vi "Append Table to Document.vi"(0 "PDF Report IN":refnum<class "PDF Report Class.lvclass">, 1 "Table properties":T18={"Table position"=1, "SpacingBefore (points)"=12.0, "SpacingAfter (points)"=12.0} {"Table position" items=["LEFT", "CENTER", "RIGHT"]}, 3 "Row background color":T20={"color"=16777225, "at each"=0}, 7 "PDF Table":refnum<class "Pdfp Table Class.lvclass">, 9 "Caption":string, 11 "error in (no error)":errorcluster, 12 "Row  [ ]":T1) -> (4 "PDF Report OUT":refnum<class "PDF Report Class.lvclass">, 15 "error out":errorcluster)   [LabVIEW 2019]
doc: "<B>ENGLISH</B>\nAppends a table to the PDF document.\n\n<B>FRANÇAIS</B>\nAjoute un tableau au document PDF.\n\nVersion 2.0\nDeveloped by Jean-Marc Simard\nCopyright © 2012, Exaprom Inc.\nAll rights reserved.\nLicense: BSD\n\nWith iTextSharp 4.1.6 (http://itextsharp.sourceforge.net)\nunder Mozilla Public License Version 1.1\n(http://www.mozilla.org/MPL/MPL-1.1.html)"
uses:
  <userlib>/Exaprom PDF/LV Class/PDF Report Class/PDF Report Class.lvclass
  <userlib>/Exaprom PDF/Controls/Table Controls/Row Back Ground color Datas.ctl
  <userlib>/Exaprom PDF/Controls/Table Controls/Table properties.ctl
  <userlib>/Exaprom PDF/Controls/Table Controls/Table position.ctl
  <userlib>/Exaprom PDF/LV Class/Pdfp Table Class/Pdfp Table Class.lvclass
  <userlib>/Exaprom PDF/Controls/Table Controls/Table Appearance and Font Row [ ].ctl
  <userlib>/Exaprom PDF/Controls/Table Controls/One Row Appearance.ctl
  <userlib>/Exaprom PDF/Controls/Table Controls/Row from to.ctl
  <userlib>/Exaprom PDF/Controls/Table Controls/Cell, Alignment, LS and Font - hide Vmerge.ctl
  <userlib>/Exaprom PDF/Controls/Table Controls/Cell Type, Alignment and LS.ctl
  <userlib>/Exaprom PDF/Controls/Table Controls/Cell Alignment 20px.ctl
  <userlib>/Exaprom PDF/Controls/Table Controls/Text vertical arrangement.ctl
  <userlib>/Exaprom PDF/Controls/Text Controls/Line spacing.ctl
  <userlib>/Exaprom PDF/Controls/Table Controls/Cell Appearance.ctl
  <userlib>/Exaprom PDF/Controls/Table Controls/Cell Border 20 px.ctl
  <userlib>/Exaprom PDF/Controls/Table Controls/Merge Horizontal.ctl
  <userlib>/Exaprom PDF/Controls/Table Controls/Merge Vertical.ctl
  <userlib>/Exaprom PDF/Controls/Font Controls/Font complete cluster.ctl
  <userlib>/Exaprom PDF/Controls/Font Controls/Font size.ctl
  <userlib>/Exaprom PDF/Controls/Font Controls/Font color.ctl
  <userlib>/Exaprom PDF/Controls/Font Controls/Type and encoding.ctl
  <userlib>/Exaprom PDF/Controls/Text Controls/Unicode/Type and run direction.ctl
  <userlib>/Exaprom PDF/Not  in the library/Images for controls/Image or Table.ctl
  C:/Program Files/National Instruments/LabVIEW 2019/user.lib/Exaprom PDF/DLL/itextsharp.dll
  DLL/itextsharp.dll
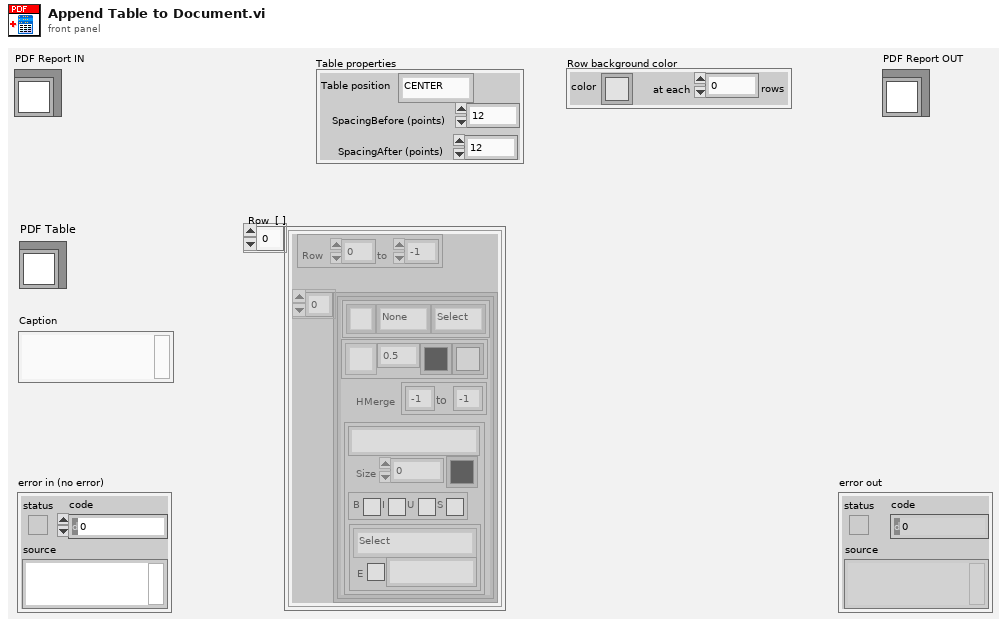
[diagram p1: front panel]
types:
  T1 = typedef "Table Appearance and Font Row [ ].ctl" = T2[]
  T2 = typedef "One Row Appearance.ctl" = cluster{"Row":T3, "Cell [ ]":T4[]}
  T3 = typedef "Row from to.ctl" = cluster{"From #":i16, "to #":i16}
  T4 = typedef "Cell, Alignment, LS and Font - hide Vmerge.ctl" = cluster{"Text":T5, "Cell Appearance":T9, "HMerge":T11, "VMerge":T12, "Font":T13}
  T5 = typedef "Cell Type, Alignment and LS.ctl" = cluster{"Cell Alignment":T6, "Text rotation":T7, "Line spacing":T8}
  T6 = typedef "Cell Alignment 20px.ctl" = u16
  T7 = typedef "Text vertical arrangement.ctl" = enum16{"None", "Clockwise", "Counterclockwise"}
  T8 = typedef "Line spacing.ctl" = enum16{"Select", "1.0", "1.5", "2.0"}
  T9 = typedef "Cell Appearance.ctl" = cluster{"Border":T10, "Thickness":sgl, "Color":u32, "BG":u32}
  T10 = typedef "Cell Border 20 px.ctl" = u16
  T11 = typedef "Merge Horizontal.ctl" = cluster{"From":i8, "to":i8}
  T12 = typedef "Merge Vertical.ctl" = cluster{"From":i8, "to":i8}
  T13 = typedef "Font complete cluster.ctl" = cluster{"Name":string, "Size":T14, "Color":T15, "Style":cluster{"Bold":bool, "Italic":bool, "Underline":bool, "Strikeout":bool}, "Type":T16}
  T14 = typedef "Font size.ctl" = sgl
  T15 = typedef "Font color.ctl" = u32
  T16 = typedef "Type and encoding.ctl" = cluster{"Type&direction":T17, "Embedded":bool, "Encoding":string}
  T17 = typedef "Type and run direction.ctl" = enum16{"Select", "ASCII", "UTF-16", "UTF-16 (default)", "UTF-16 (LTR)", "UTF-16 (RTL)"}
  T18 = typedef "Table properties.ctl" = cluster{"Table position":T19, "SpacingBefore (points)":sgl, "SpacingAfter (points)":sgl}
  T19 = typedef "Table position.ctl" = i32
  T20 = typedef "Row Back Ground color Datas.ctl" = cluster{"color":u32, "at each":i16}
  T21 = typedef "Image or Table.ctl" = enum16{"Image", "Table"}
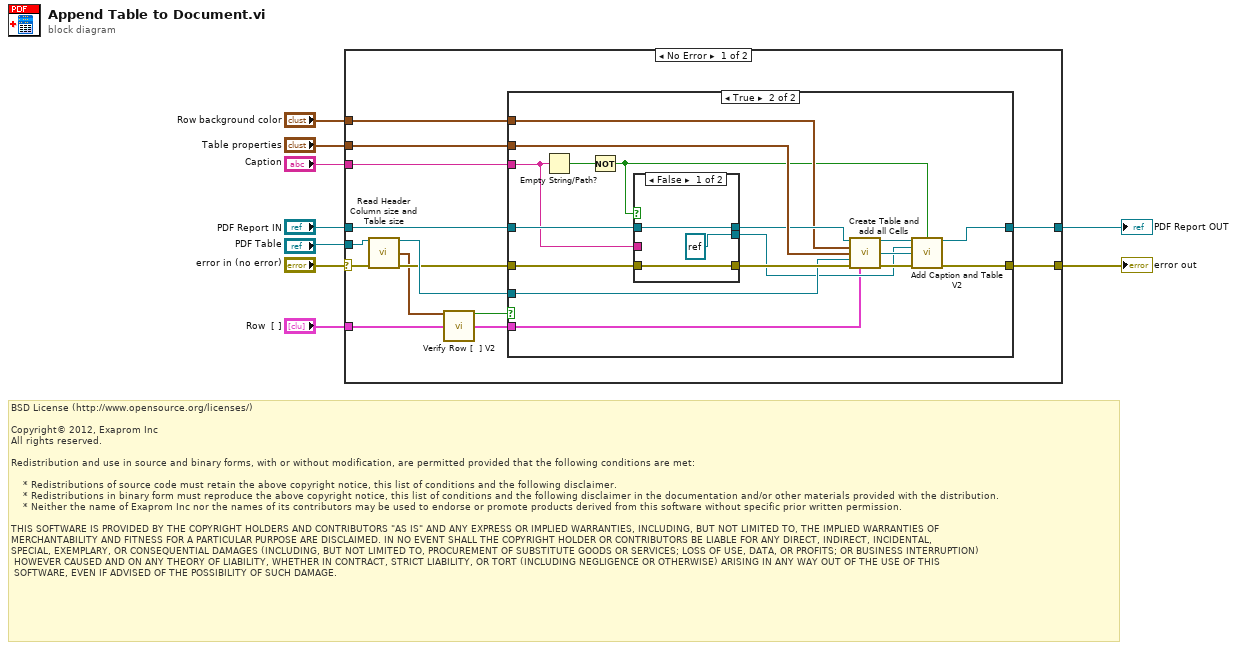
[diagram p0: block diagram]
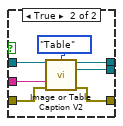
[diagram p3: hidden frame]
diagram:
  # "BSD License (http://www.opensource.org/licenses/)\n\nCopyright© 2012, Exaprom Inc\nAll rights reserved.\n\nRedistribution and use in source and binary forms, with or without modification, are permitted provided that the following conditions are met:\n\n    * Redistributions of source code must retain the above copyright notice, this list of conditions and the following disclaimer.\n    * Redistributions in binary form must reproduce the above copyright notice, this list of conditions and the following disclaimer in the documentation and/or other materials provided with the distribution.\n    * Neither the name of Exaprom Inc nor the names of its contributors may be used to endorse or promote products derived from this software without specific prior written permission.\n\nTHIS SOFTWARE IS PROVIDED BY THE COPYRIGHT HOLDERS AND CONTRIBUTORS \"AS IS\" AND ANY EXPRESS OR IMPLIED WARRANTIES, INCLUDING, BUT NOT LIMITED TO, THE IMPLIED WARRANTIES OF \nMERCHANTABILITY AND FITNESS FOR A PARTICULAR PURPOSE ARE DISCLAIMED. IN NO EVENT SHALL THE COPYRIGHT HOLDER OR CONTRIBUTORS BE LIABLE FOR ANY DIRECT, INDIRECT, INCIDENTAL,\nSPECIAL, EXEMPLARY, OR CONSEQUENTIAL DAMAGES (INCLUDING, BUT NOT LIMITED TO, PROCUREMENT OF SUBSTITUTE GOODS OR SERVICES; LOSS OF USE, DATA, OR PROFITS; OR BUSINESS INTERRUPTION)\n HOWEVER CAUSED AND ON ANY THEORY OF LIABILITY, WHETHER IN CONTRACT, STRICT LIABILITY, OR TORT (INCLUDING NEGLIGENCE OR OTHERWISE) ARISING IN ANY WAY OUT OF THE USE OF THIS\n SOFTWARE, EVEN IF ADVISED OF THE POSSIBILITY OF SUCH DAMAGE."
  n1 = case shown="No Error" "error in (no error)" {
    selector: "error in (no error)" -> [w17 w53]
    tunnel: "Table properties" -> [w22 _]
    tunnel: "PDF Report IN" -> [w23 w54]
    tunnel: "Caption" -> [w18 _]
    tunnel: "Row background color" -> [w21 _]
    tunnel: [w19 w54] -> w4
    tunnel: [w20 w53] -> w3
    tunnel: "PDF Table" -> [w16 _]
    tunnel: "Row  [ ]" -> [w12 _]
    frame No Error {
      n2 = call-dynamic "Read Header Column size and Table size.vi"("Pdfp Table Class in"=w16, "error in (no error)"=w17) -> ("Pdfp Table Class out"=w15:refnum<class "Pdfp Table Class.lvclass">, "Table size"=w11:cluster{"# Column":u16, "# Row":u16}, "error out"=w14:errorcluster)  [unwired: 9 in, 2 out]
      n3 = call <userlib>:"Verify Row [  ] V2.vi"("Table size"=w11, "Row  [ ] IN"=w12) -> ("Create Table?"=w10:bool, "Row  [ ] OUT"=w13:T1)  [unwired: 12 in]
      n4 = case shown="True" w10 {
        tunnel: w14 -> [w25 w42]
        tunnel: w23 -> [w24 w41]
        tunnel: w15 -> [_ w39]
        tunnel: w22 -> [_ w38]
        tunnel: w21 -> [_ w36]
        tunnel: [w25 w35] -> w20
        tunnel: [w24 w34] -> w19
        tunnel: w18 -> [_ w31]
        tunnel: w13 -> [_ w26]
        frame False {
        }
        frame True {
          n5 = Empty String/Path?(string/path=w31) -> (empty?=w28:bool)
          n6 = Not(x=w28) -> (.not. x?=w27:bool)
          n7 = case shown="False" w27 {
            tunnel: [w45 w52] -> w37
            tunnel: w41 -> [w45 w51]
            tunnel: w31 -> [_ w50]
            tunnel: [w44 w49] -> w40
            tunnel: [refnum<k24> refnum ("Paragraph Refnum") w48] -> w29
            tunnel: w42 -> [w44 w47]
            frame False {
              (unwired) sgl 2.0 ("Largeur (default unit)")
              (unwired) u32 0
              (unwired) refnum<k24> refnum ("Cell ref")
              (unwired) sgl 0.0 ("TotalHeight")
            }
            frame True {
              n8 = call <userlib>:"Image or Table Caption V2.vi"("PDF Report IN"=w51, "Image or Table"=Image_or_Table."Table", "Caption IN"=w50, "error IN"=w47) -> ("PDF Report OUT"=w52:refnum<class "PDF Report Class.lvclass">, "PdfpTable Refnum"=w48:refnum<k24>, "error OUT"=w49:errorcluster)  [unwired: 4 in, 5 out]
            }
          }
          n9 = call <userlib>:"Create Table and add all Cells.vi"("PDF Report IN"=w37, "Row background color"=w36, "Table properties"=w38, "PDF Table"=w39, "error in (no error)"=w40, "Row  [ ]"=w26) -> ("PDF Report OUT"=w33:refnum<class "PDF Report Class.lvclass">, "PdfPTable"=w30:refnum<k24>, "error out"=w32:errorcluster)  [unwired: 7 in]
          n10 = call <userlib>:"Add Caption and Table V2.vi"("PDF Report IN"=w33, "Caption?"=w27, "PdfpTable Title Refnum"=w29, "PdfPTable"=w30, "error in (no error)"=w32) -> ("PDF Report OUT"=w34:refnum<class "PDF Report Class.lvclass">, "error out"=w35:errorcluster)  [unwired: 9 out]
        }
      }
    }
    frame Error {
    }
  }
  "error out" <- w3
  "PDF Report OUT" <- w4
